vi "Draw_Img_Center.vi"(6 "[IN] Color":u32(colorbox)=16711680, 8 "error IN":errorcluster, 11 "[IN] Image":T1) -> (0 "error OUT":errorcluster, 3 "[OUT] Image":T1)   [LabVIEW 2020]
uses:
  <vilib>/vision/Image Controls.llb/IMAQ Image.ctl
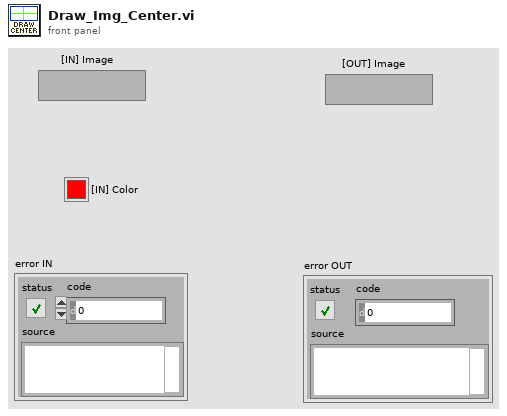
[diagram p1: front panel]
types:
  T1 = typedef "IMAQ Image.ctl" = refnum<image>
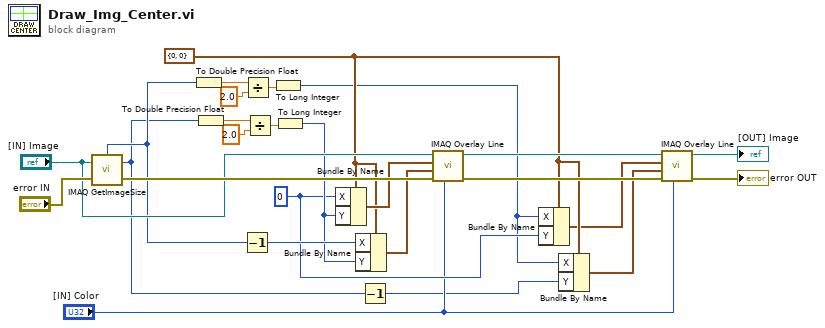
[diagram p0: block diagram]
diagram:
  w7 = 0 ("X")
  w8 = cluster{"X":i32, "Y":i32} {"X"=0, "Y"=0} ("Start Point")
  n1 = call "IMAQ GetImageSize"("Image"="[IN] Image", "error in (no error)"="error IN") -> ("Y Resolution"=w2:i32, "X Resolution"=w15:i32, "error out"=w25:errorcluster)  [unwired: 2 in]
  n2 = To Double Precision Float(number=w15) -> (double precision float=w18:dbl)
  n3 = To Double Precision Float(number=w2) -> (double precision float=w23:dbl)
  n4 = Decrement(x=w15) -> (x-1=w14:i32)
  n5 = Divide(x=w18, y=2.0) -> (x/y=w16:dbl)
  n6 = Divide(x=w23, y=2.0) -> (x/y=w21:dbl)
  n7 = To Long Integer(number=w16) -> (32bit integer=w6:i32)
  n8 = To Long Integer(number=w21) -> (32bit integer=w13:i32)
  n9 = Bundle By Name(cluster=w8, "X"=w7, "Y"=w13) -> (w20:cluster{"X":i32, "Y":i32})
  n10 = Bundle By Name(cluster=w8, "X"=w14, "Y"=w13) -> (w19:cluster{"X":i32, "Y":i32})
  n11 = Decrement(x=w2) -> (x-1=w1:i32)
  n12 = call "IMAQ Overlay Line"("Color"="[IN] Color", "error in (no error)"=w25, "End Point"=w19, "Start Point"=w20, "Image"="[IN] Image") -> ("error out"=w12:errorcluster, "Image Out"=w11:T1)  [unwired: 5 in]
  n13 = Bundle By Name(cluster=w8, "X"=w6, "Y"=w7) -> (w5:cluster{"X":i32, "Y":i32})
  n14 = Bundle By Name(cluster=w8, "X"=w6, "Y"=w1) -> (w4:cluster{"X":i32, "Y":i32})
  n15 = call "IMAQ Overlay Line"("Color"="[IN] Color", "error in (no error)"=w12, "End Point"=w4, "Start Point"=w5, "Image"=w11) -> ("error out"=→"error OUT":errorcluster, "Image Out"=→"[OUT] Image":T1)  [unwired: 5 in]
